vi "Set secondaryContainer.vi"(8 "error in":errorcluster, 10 "secondaryContainer":u32(colorbox), 11 "Material-Scheme in":refnum<class "Material-Scheme.lvclass">) -> (0 "error out":errorcluster, 3 "Material-Scheme out":refnum<class "Material-Scheme.lvclass">)   [LabVIEW 2021, in "TSC Material Theme.lvlib" / "Material-Scheme.lvclass"]
uses:
  Material-Scheme.lvclass
  Material-Scheme.lvclass/Material-Scheme.ctl
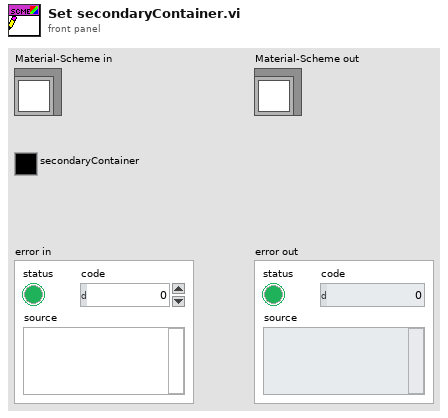
[diagram p1: front panel]
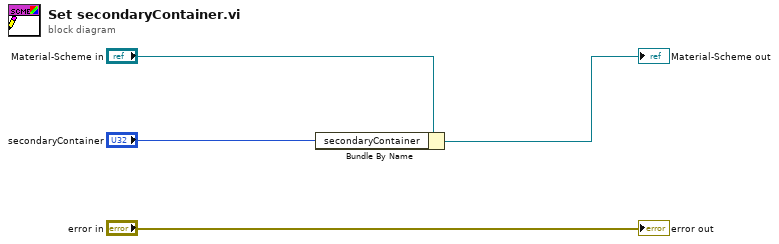
[diagram p0: block diagram]
diagram:
  n1 = Bundle By Name(cluster="Material-Scheme in", "secondaryContainer"="secondaryContainer") -> (→"Material-Scheme out":refnum<class "Material-Scheme.lvclass">)
  "error out" <- "error in"
